vi "Generate Instructions.vi"(0 "State":T1=enum."Stagger Stop", 1 "Wall Left?":bool=TRUE, 2 "dt":dbl=100.0, 3 "Target Distance":dbl=250.0) -> (7 "Target Angle":dbl=0.008343690621517926)   [LabVIEW 2017]
uses:
  state-manager/State.ctl
  Globals/Pose.vi
  Globals/Motor Speed Multiplier.vi
panel:
  out "Ramp Initial Wall Distance":dbl=-179.11363508234209
  in  "Limit for Hitting Wall (mm)":dbl=350.0 format="%#_13g"
  in  "Minimum Magnitude":dbl
  in  "Size of Array":i32=20
  in  "Maximum Angle (deg)":dbl=10.0
  in  "Minimum Angle (deg)":dbl=-10.0
  # "STAGGER STOP PARAMETERS"
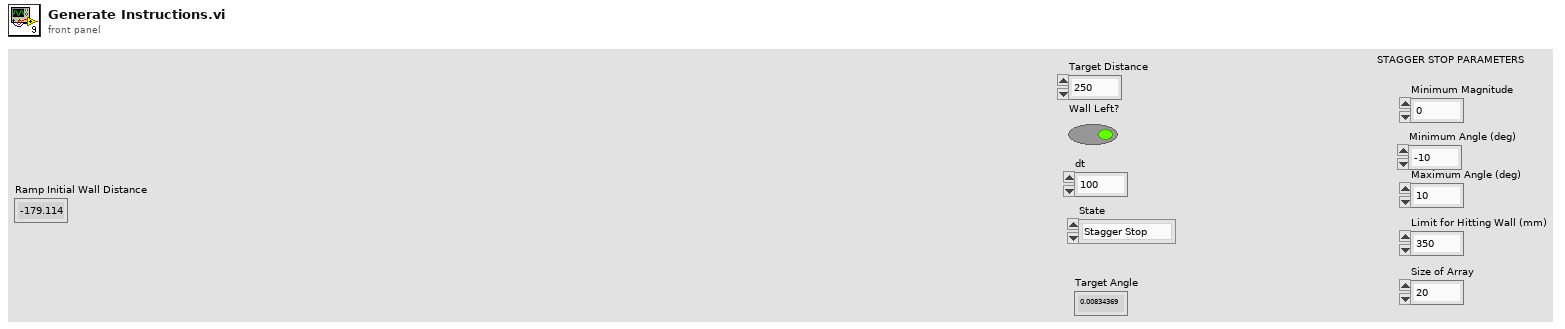
[diagram p1: front panel]
types:
  T1 = typedef "State.ctl" = enum16{"Wait", "Recenter", "Follow Wall", "Zig Zag", "Ramp", "Cross Rough Terrain", "Stagger Stop", "Obstacle Avoidance"}
  T2 = cluster{"Lidar Magnitudes":dbl[], "Lidar Directions":dbl[]}
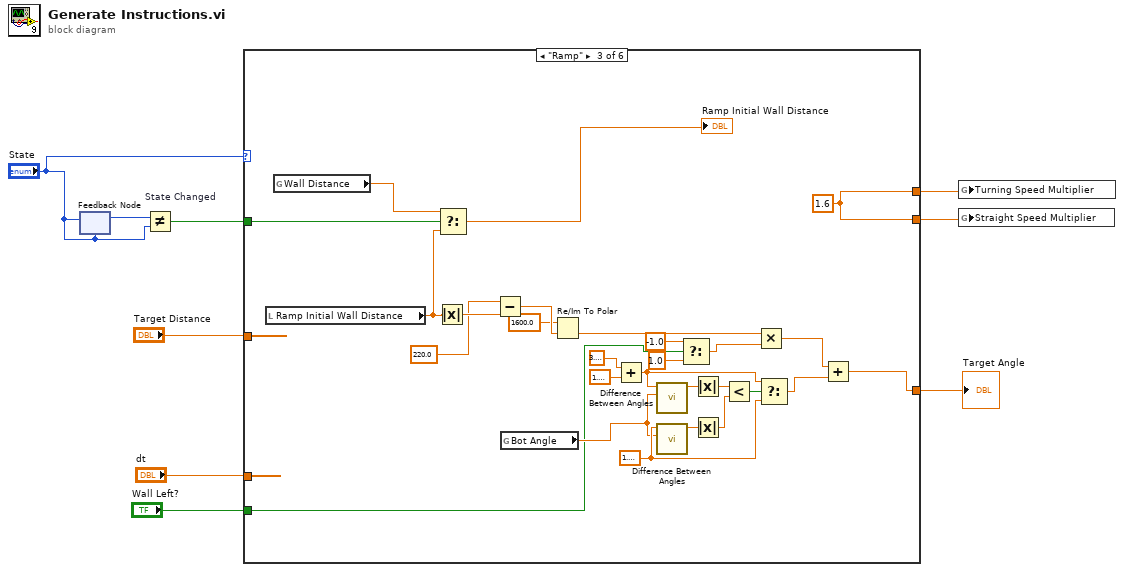
[diagram p0: block diagram]
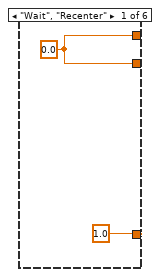
[diagram p2: hidden frame]
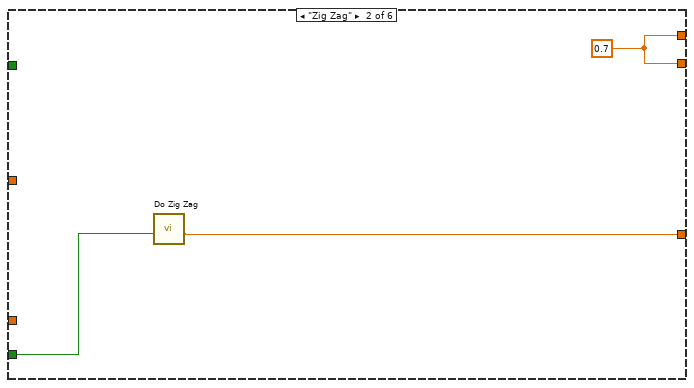
[diagram p3: hidden frame]
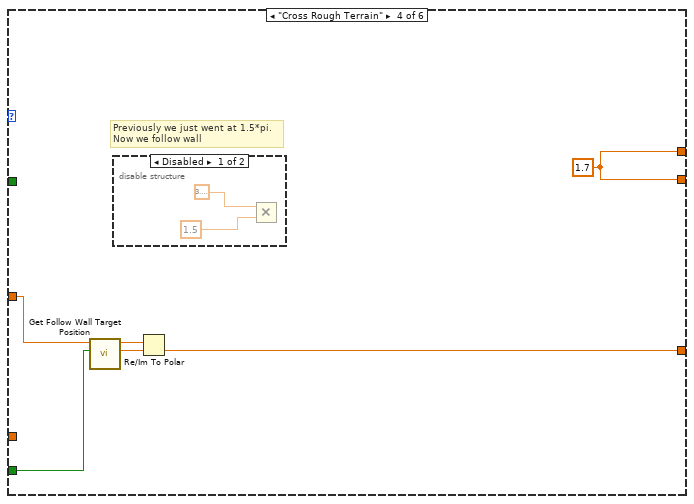
[diagram p4: hidden frame]
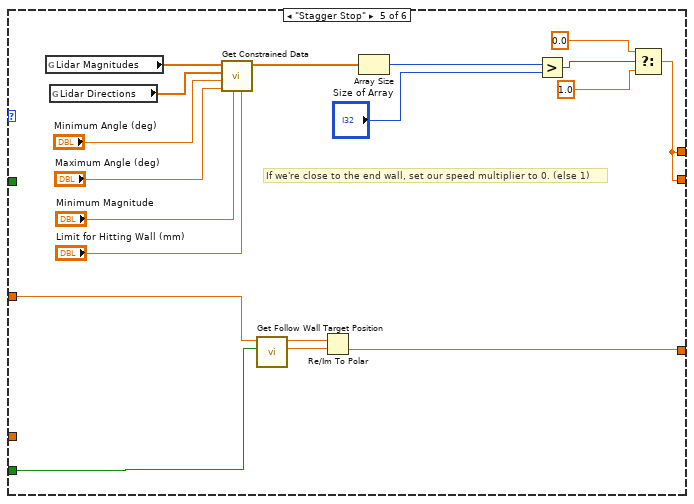
[diagram p6: hidden frame]
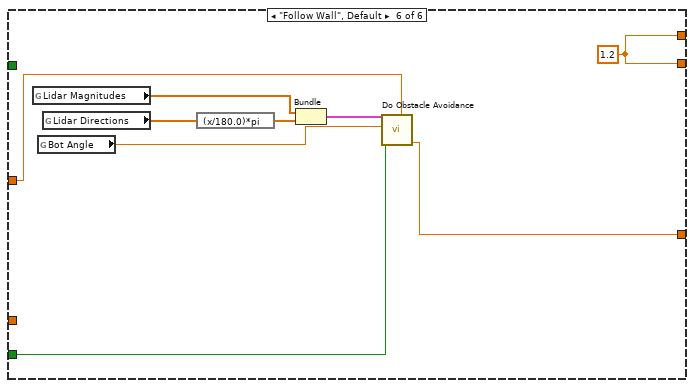
[diagram p7: hidden frame]
diagram:
  n1 = feedback #1("State") -> (w3:T1)
  n2 = feedback-in #1("State") -> ()
  n3 = Not Equal? "State Changed"(x=w3, y="State") -> (x != y?=w1:bool)
  n4 = case shown="\"Ramp\"" "State" {
    tunnel: [w10 w14 w32 w42 w50 w68] -> w7
    tunnel: [w10 w14 w32 w42 w50 w68] -> w8
    tunnel: "dt" -> [_ _ _ _ _ _]
    tunnel: "Target Distance" -> [_ _ _ w47 w53 w70]
    tunnel: [1.0 w12 w24 w43 w51 w69] -> w4
    tunnel: "Wall Left?" -> [_ w13 w19 w46 w52 w71]
    tunnel: w1 -> [_ _ w31 _ _ _]
    frame "Wait", "Recenter" {
      w10 = 0.0
    }
    frame "Zig Zag" {
      w14 = 0.7
      n5 = call "Do Zig Zag.vi"("Wall Left?"=w13) -> ("Target Angle"=w12:dbl)  [unwired: 10 in]
    }
    frame "Ramp" {
      w33 = 1.5707963267948966
      w32 = 1.6
      n6 = local read "Ramp Initial Wall Distance"() -> (w28:dbl)
      n7 = global read "Pose.vi" "Wall Distance"() -> (w30:dbl)
      n8 = Absolute Value(x=w28) -> (abs(x)=w27:dbl)
      n9 = Select(t=w30, s=w31, f=w28) -> (s? t:f=→"Ramp Initial Wall Distance":dbl)
      n10 = Subtract(x=220.0, y=w27) -> (x-y=w23:dbl)
      n11 = global read "Pose.vi" "Bot Angle"() -> (w26:dbl)
      n12 = Re/Im To Polar(2:w23, 3:1600.0 ("x")) -> (0:w20:dbl)  [unwired: 1 out]
      n13 = Add(x=3.141592653589793, y=1.5707963267948966) -> (x+y=w34:dbl)
      n14 = call "Difference Between Angles.vi"("Angle 2"=w26, "Angle 1"=w34) -> ("Difference"=w39:dbl)  [unwired: 9 in]
      n15 = call "Difference Between Angles.vi"("Angle 2"=w26, "Angle 1"=w33) -> ("Difference"=w38:dbl)  [unwired: 9 in]
      n16 = Select(t=-1.0, s=w19, f=1.0) -> (s? t:f=w16:dbl)
      n17 = Absolute Value(x=w39) -> (abs(x)=w36:dbl)
      n18 = Absolute Value(x=w38) -> (abs(x)=w35:dbl)
      n19 = Less?(x=w36, y=w35) -> (x < y?=w37:bool)
      n20 = Multiply(x=w20, y=w16) -> (x*y=w15:dbl)
      n21 = Select(t=w34, s=w37, f=w33) -> (s? t:f=w25:dbl)
      n22 = Add(x=w15, y=w25) -> (x+y=w24:dbl)
    }
    frame "Cross Rough Terrain" {
      w42 = 1.7
      # "Previously we just went at 1.5*pi.\nNow we follow wall"
      n23 = call "Get Follow Wall Target Position.vi"("Wall left?"=w46, "Target Distance"=w47) -> ("Target Y (Relative)"=w45:dbl, "Target X (Relative)"=w44:dbl)  [unwired: 6 in]
      n24 = disable-structure shown="Disabled" {
        frame Disabled {
          n25 = Multiply(x=3.141592653589793, y=1.5) -> ()  [unwired: 1 out]
        }
        frame Enabled {
        }
      }
      n26 = Re/Im To Polar(2:w45, 3:w44) -> (0:w43:dbl)  [unwired: 1 out]
    }
    frame "Stagger Stop" {
      # "If we're close to the end wall, set our speed multiplier to 0. (else 1)"
      n27 = global read "Pose.vi" "Lidar Magnitudes"() -> (w66:dbl[])
      n28 = global read "Pose.vi" "Lidar Directions"() -> (w65:dbl[])
      n29 = call "Get Constrained Data.vi"("Maximum Magnitude"="Limit for Hitting Wall (mm)", "Minimum Magnitude"="Minimum Magnitude", "Maximum Angle (rad)"="Maximum Angle (deg)", "Minimum Angle (rad)"="Minimum Angle (deg)", "Lidar Directions (rad)"=w65, "Lidar Magnitudes"=w66) -> ("Constrained Magnitudes"=w56:dbl[])  [unwired: 4 in, 1 out]
      n30 = call "Get Follow Wall Target Position.vi"("Wall left?"=w52, "Target Distance"=w53) -> ("Target Y (Relative)"=w54:dbl, "Target X (Relative)"=w55:dbl)  [unwired: 6 in]
      n31 = Re/Im To Polar(2:w54, 3:w55) -> (0:w51:dbl)  [unwired: 1 out]
      n32 = Array Size(array=w56) -> (size(s)=w62:i32)
      n33 = Greater?(x=w62, y="Size of Array") -> (0:w60:bool)
      n34 = Select(t=0.0, s=w60, f=1.0) -> (s? t:f=w50:dbl)
    }
    frame "Follow Wall", Default {
      w68 = 1.2
      n35 = global read "Pose.vi" "Lidar Magnitudes"() -> (w76:dbl[])
      n36 = global read "Pose.vi" "Bot Angle"() -> (w74:dbl)
      n37 = global read "Pose.vi" "Lidar Directions"() -> (w73:dbl[])
      n38 = expression code="(x/180.0)*pi" ("degrees to radians")(w73) -> (w72:dbl[])
      n39 = Bundle("Lidar Magnitudes"=w76, "Lidar Directions"=w72) -> (w75:T2)  [unwired: 1 in]
      n40 = call "Do Obstacle Avoidance.vi"("Target Distance"=w70, "Wall Left?"=w71, "Bot Angle (rad)"=w74, "Lidar Data (mm, rad)"=w75) -> ("Target Angle"=w69:dbl)  [unwired: 7 in]
    }
  }
  "Target Angle" <- w4
  n41 = global write "Motor Speed Multiplier.vi" "Turning Speed Multiplier"(w7) -> ()
  n42 = global write "Motor Speed Multiplier.vi" "Straight Speed Multiplier"(w8) -> ()
